vi "Get TDC Info.vi"(8 "error in (no error)":errorcluster, 10 "Card no.":i32, 11 "TDCManager":T2) -> (0 "error out":errorcluster, 2 "TDC Info":T1, 3 "TDCManager":T2)   [LabVIEW 2016, in "HPTDC Driver Library.lvlib"]
uses:
  HPTDC Driver Library.lvlib
  Typedefs/TDCManager.ctl
  C:/Users/CRT Controller/CRTC Labview Application/Source/HPTDC Driver Library Folder/Library files/hptdc_net4_3.7.0_x64.dll
  hptdc_net4_3.7.0_x64.dll
  Typedefs/HPTDCInfo.ctl
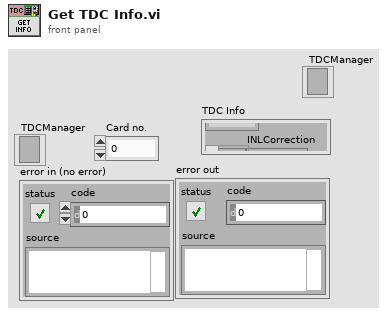
[diagram p1: front panel]
types:
  T1 = typedef "HPTDC Driver Library.lvlib/HPTDCInfo.ctl" = cluster{"boardConfiguration":u8, "bufferSize":i32, "channelCount":i32, "channelStart":i32, "DNLData":i16[], "fifoSize":i32, "flashValid":bool, "highResChannelCount":i32, "highResChannelStart":i32, "index":i32, "INLCorrection":i32[], "lowResChannelCount":i32, "lowResChannelStart":i32, "resolution":dbl, "serialNumber":i32, "version":i32}
  T2 = typedef "HPTDC Driver Library.lvlib/TDCManager.ctl" = refnum<k24>
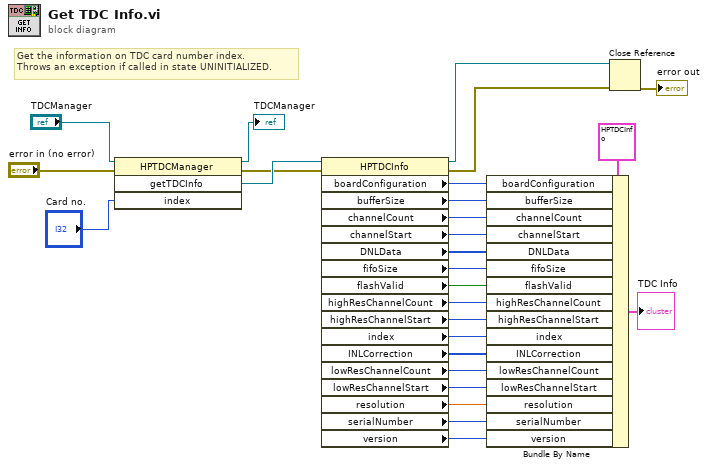
[diagram p0: block diagram]
diagram:
  # "Get the information on TDC card number index.\nThrows an exception if called in state UNINITIALIZED."
  n1 = invoke class="HPTDCManager" method="getTDCInfo"(reference="TDCManager", error in="error in (no error)", "index"="Card no.") -> (reference out=→"TDCManager":T2, error out=w23:errorcluster, "getTDCInfo"=w24:refnum<k24>)  [unwired: 1 in, 1 out]
  n2 = property class="HPTDCInfo"(reference=w24, error in=w23) -> (reference out=w4:refnum<k24>, error out=w5:errorcluster, "boardConfiguration"=w21:u8, "bufferSize"=w20:i32, "channelCount"=w19:i32, "channelStart"=w18:i32, "DNLData"=w17:i16[], "fifoSize"=w16:i32, "flashValid"=w15:bool, "highResChannelCount"=w14:i32, "highResChannelStart"=w13:i32, "index"=w12:i32, "INLCorrection"=w11:i32[], "lowResChannelCount"=w10:i32, "lowResChannelStart"=w9:i32, "resolution"=w8:dbl, "serialNumber"=w7:i32, "version"=w6:i32)
  n3 = Bundle By Name(cluster=T1 {"boardConfiguration"=0, "bufferSize"=0, "channelCount"=0, "channelStart"=0, "DNLData"=[], "fifoSize"=0, "flashValid"=FALSE, "highResChannelCount"=0, "highResChannelStart"=0, "index"=0, "INLCorrection"=[], "lowResChannelCount"=0, "lowResChannelStart"=0, "resolution"=0.0, "serialNumber"=0, "version"=0}, "boardConfiguration"=w21, "bufferSize"=w20, "channelCount"=w19, "channelStart"=w18, "DNLData"=w17, "fifoSize"=w16, "flashValid"=w15, "highResChannelCount"=w14, "highResChannelStart"=w13, "index"=w12, "INLCorrection"=w11, "lowResChannelCount"=w10, "lowResChannelStart"=w9, "resolution"=w8, "serialNumber"=w7, "version"=w6) -> (→"TDC Info":T1)
  n4 = Close Reference(reference=w4, error in (no error)=w5) -> (error out=→"error out":errorcluster)
